vi "niRFUtil WFM Resample (complex wfm).vi"(0 "Complex Waveform In":T1 {"y" format="%.2f"; "dx" format="%^.2e"; "x0" format="%^.2e"}, 5 "Desired Sample Rate (Hz)":dbl=1.0 format="%^.3e", 11 "error in (no error)":errorcluster, 12 "Allowable Sampling Rate Error (ppm)":dbl=1.0 format="%.2g") -> (4 "Complex Waveform Out":T1 {"y" format="%.2f"; "dx" format="%^.2e"; "x0" format="%^.2e"}, 15 "error out":errorcluster)   [LabVIEW 2015, in "niRFUtil.lvlib"]
uses:
  niRFUtil.lvlib
  Includes/niRFUtil INC Complex Waveform.ctl
  Includes/niRFUtil INC Complex Array.ctl
  Filters, Transforms, Windows/niRFUtil FTW Decimating FIR Filter (complex wfm).vi
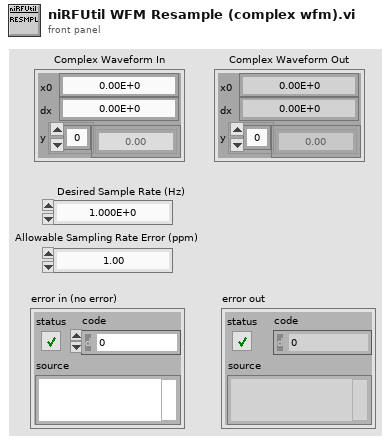
[diagram p1: front panel]
types:
  T1 = typedef "niRFUtil.lvlib/niRFUtil INC Complex Waveform.ctl" = cluster{"x0":dbl, "dx":dbl, "y":T2}
  T2 = typedef "niRFUtil.lvlib/niRFUtil INC Complex Array.ctl" = csg[]
  T3 = typedef "niRFUtil.lvlib/niRFUtil INC Real Waveform.ctl" = cluster{"x0":dbl, "dx":dbl, "y":T4}
  T4 = typedef "niRFUtil.lvlib/niRFUtil INC Real Array.ctl" = sgl[]
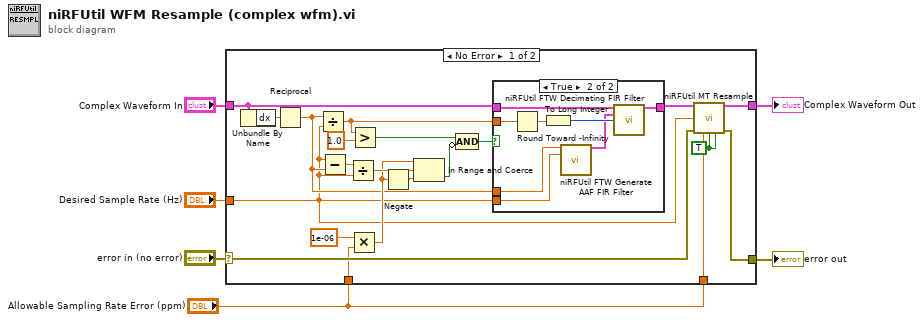
[diagram p0: block diagram]
diagram:
  n1 = case shown="No Error" "error in (no error)" {
    selector: "error in (no error)" -> [w23 w38]
    tunnel: "Complex Waveform In" -> [w26 w37]
    tunnel: [w25 w38] -> w5
    tunnel: [w24 w37] -> w4
    tunnel: "Desired Sample Rate (Hz)" -> [w12 _]
    tunnel: "Allowable Sampling Rate Error (ppm)" -> [w19 _]
    tunnel: "Allowable Sampling Rate Error (ppm)" -> [w8 _]
    frame No Error {
      w7 = TRUE ("flush buffers? (F)")
      n2 = Unbundle By Name(w26) -> ("dx"=w27:dbl)
      n3 = Reciprocal(x=w27) -> (1/x=w13:dbl)
      n4 = Divide(x=w13, y=w12) -> (x/y=w20:dbl)
      n5 = Subtract(x=w12, y=w13) -> (x-y=w18:dbl)
      n6 = Divide(x=w18, y=w12) -> (x/y=w17:dbl)
      n7 = Multiply(x=1e-06, y=w8) -> (x*y=w14:dbl)
      n8 = Greater?(x=w20, y=1.0) -> (0:w10:bool)
      n9 = Negate(x=w14) -> (-x=w15:dbl)
      n10 = In Range and Coerce(upper limit=w14, x=w17, lower limit=w15) -> (In Range?=w11:bool)  [unwired: 1 out]
      n11 = Compound Arithmetic op=AND(w10, invert w11) -> (w9:bool)
      n12 = case shown="True" w9 {
        tunnel: w26 -> [w28 w33]
        tunnel: [w28 w36] -> w22
        tunnel: w20 -> [_ w32]
        tunnel: w12 -> [_ w29]
        tunnel: w13 -> [_ w30]
        frame False {
        }
        frame True {
          n13 = Round Toward -Infinity(1:w32) -> (0:w35:dbl)
          n14 = To Long Integer(number=w35) -> (32bit integer=w34:i32)
          n15 = call "niRFUtil FTW Generate AAF FIR Filter.vi"("Input Sample Rate (Hz)"=w30, "Desired Sample Rate (Hz)"=w29) -> ("Anti Alias Filter"=w31:T3)  [unwired: 13 in]
          n16 = call-poly "niRFUtil FTW Decimating FIR Filter.vi"("Waveform In"=w33, "Filter"=w31, "Decimating Factor"=w34) -> ("Waveform Out"=w36:T1)  [unwired: 12 in]
        }
      }
      n17 = call "niRFUtil MT Resample.vi"("Waveform In"=w22, "desired sample rate (Hz)"=w12, "error in (no error)"=w23, "allowable sample rate error (ppm)"=w19, "reset? (T)"=w7, "flush buffers? (F)"=w7) -> ("Waveform Out"=w24:T1, "error out"=w25:errorcluster)  [unwired: 8 in]
    }
    frame Error {
    }
  }
  "Complex Waveform Out" <- w4
  "error out" <- w5
